vi "SwerveMain.vi"   [LabVIEW 2018]
uses:
  <vilib>/Rock Robotics/WPI/ThirdParty/Phoenix-LabVIEW/Motor Controller/Controls/CTRE_Phoenix_MotorControl_ControlMode.ctl
  <vilib>/Rock Robotics/Network Tables/NT Read Numeric Array.vi
  <vilib>/Rock Robotics/Network Tables/NT Write Numeric Array.vi
types:
  T1 = typedef "WPI_MotorControlDeviceRef.ctl" = cluster{"DeviceStatus":errorcluster, "Type":T2, "PWM":cluster{"PWM Channel":T3, "DeadBand":T4}, "CAN":cluster{"Device Number":u8, "SetOutput VI Ref":variant, "GetOutput VI Ref":variant, "Enable VI Ref":variant, "Disable VI Ref":variant, "Data":variant}, "Invert":bool, "DIO PWM":cluster{"PWM \"Enable\" Channel":T3, "DIOChannel":T5, "PWM Rate":dbl}}
  T2 = typedef "WPI_MotorControlType.ctl" = enum16{"PWM", "CAN", "DIO PWM"}
  T3 = typedef "FPGA_DIOPWMChannel.ctl" = enum8{"PWM 0", "PWM 1", "PWM 2", "PWM 3", "PWM 4", "PWM 5", "PWM 6", "PWM 7", "PWM 8", "PWM 9", "PWM MXP 0", "PWM MXP 1", "PWM MXP 2", "PWM MXP 3", "PWM MXP 4", "PWM MXP 5", "PWM MXP 6", "PWM MXP 7", "PWM MXP 8", "PWM MXP 9", "Invalid"}
  T4 = typedef "WPI_PWMDeadband.ctl" = cluster{"Name":string, "maxPositivePwm":i32, "minPositivePwm":i32, "centerPwm":i32, "maxNegativePwm":i32, "minNegativePwm":i32, "angularRange":u16}
  T5 = typedef "FPGA_DIOChannel.ctl" = enum8{"DIO 0", "DIO 1", "DIO 2", "DIO 3", "DIO 4", "DIO 5", "DIO 6", "DIO 7", "DIO 8", "DIO 9", "DIO MXP 0", "DIO MXP 1", "DIO MXP 2", "DIO MXP 3", "DIO MXP 4", "DIO MXP 5", "DIO MXP 6", "DIO MXP 7", "DIO MXP 8", "DIO MXP 9", "DIO MXP 10", "DIO MXP 11", "DIO MXP 12", "DIO MXP 13", "DIO MXP 14", "DIO MXP 15", "SPI Port CS1", "SPI Port CS2", "SPI Port CS3", "SPI Port MISO", "SPI Port MOSI", "Invalid"}
  T6 = typedef "WPI_AnalogChannelDevRef.ctl" = cluster{"DevStatus":errorcluster, "Analog Channel":T7}
  T7 = typedef "FPGA_AIChannel.ctl" = enum8{"AI 0", "AI 1", "AI 2", "AI 3", "AI MXP 0", "AI MXP 1", "AI MXP 2", "AI MXP 3", "Invalid"}
  T8 = cluster{"PhoenixMotorControlDevRef":T1, "PhoenixMotorControlDevRef":T1, "PhoenixMotorControlDevRef":T1, "PhoenixMotorControlDevRef":T1}
  T9 = typedef "CTRE_Phoenix_MotorControl_ControlMode.ctl" = u16
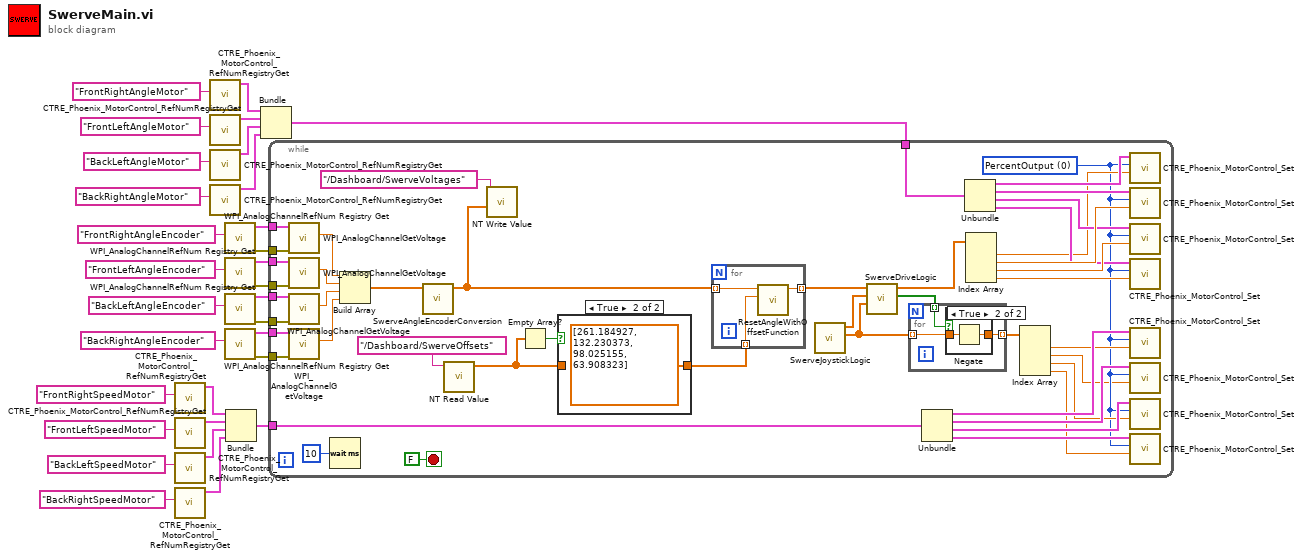
[diagram p0: block diagram]
diagram:
  n1 = call <vilib>:"CTRE_Phoenix_MotorControl_RefNumRegistryGet.vi"("refnum name"="FrontRightSpeedMotor") -> ("PhoenixMotorControlDevRef"=w8:T1)  [unwired: 9 in, 1 out]
  n2 = call <vilib>:"CTRE_Phoenix_MotorControl_RefNumRegistryGet.vi"("refnum name"="FrontLeftSpeedMotor") -> ("PhoenixMotorControlDevRef"=w16:T1)  [unwired: 9 in, 1 out]
  n3 = call <vilib>:"CTRE_Phoenix_MotorControl_RefNumRegistryGet.vi"("refnum name"="BackLeftSpeedMotor") -> ("PhoenixMotorControlDevRef"=w17:T1)  [unwired: 9 in, 1 out]
  n4 = call <vilib>:"CTRE_Phoenix_MotorControl_RefNumRegistryGet.vi"("refnum name"="BackRightSpeedMotor") -> ("PhoenixMotorControlDevRef"=w18:T1)  [unwired: 9 in, 1 out]
  n5 = call <vilib>:"CTRE_Phoenix_MotorControl_RefNumRegistryGet.vi"("refnum name"="FrontRightAngleMotor") -> ("PhoenixMotorControlDevRef"=w5:T1)  [unwired: 9 in, 1 out]
  n6 = call <vilib>:"CTRE_Phoenix_MotorControl_RefNumRegistryGet.vi"("refnum name"="FrontLeftAngleMotor") -> ("PhoenixMotorControlDevRef"=w9:T1)  [unwired: 9 in, 1 out]
  n7 = call <vilib>:"CTRE_Phoenix_MotorControl_RefNumRegistryGet.vi"("refnum name"="BackLeftAngleMotor") -> ("PhoenixMotorControlDevRef"=w10:T1)  [unwired: 9 in, 1 out]
  n8 = call <vilib>:"CTRE_Phoenix_MotorControl_RefNumRegistryGet.vi"("refnum name"="BackRightAngleMotor") -> ("PhoenixMotorControlDevRef"=w7:T1)  [unwired: 9 in, 1 out]
  n9 = call <vilib>:"WPI_AnalogChannelRefNum Registry Get.vi"("refnum name"="FrontRightAngleEncoder") -> ("error out"=w4:errorcluster, "AIDeviceRef"=w14:T6)  [unwired: 9 in]
  n10 = call <vilib>:"WPI_AnalogChannelRefNum Registry Get.vi"("refnum name"="FrontLeftAngleEncoder") -> ("error out"=w3:errorcluster, "AIDeviceRef"=w13:T6)  [unwired: 9 in]
  n11 = call <vilib>:"WPI_AnalogChannelRefNum Registry Get.vi"("refnum name"="BackLeftAngleEncoder") -> ("error out"=w2:errorcluster, "AIDeviceRef"=w12:T6)  [unwired: 9 in]
  n12 = call <vilib>:"WPI_AnalogChannelRefNum Registry Get.vi"("refnum name"="BackRightAngleEncoder") -> ("error out"=w1:errorcluster, "AIDeviceRef"=w11:T6)  [unwired: 9 in]
  n13 = Bundle("PhoenixMotorControlDevRef"=w8, "PhoenixMotorControlDevRef"=w16, "PhoenixMotorControlDevRef"=w17, "PhoenixMotorControlDevRef"=w18) -> (w15:T8)  [unwired: 1 in]
  n14 = Bundle("PhoenixMotorControlDevRef"=w5, "PhoenixMotorControlDevRef"=w9, "PhoenixMotorControlDevRef"=w10, "PhoenixMotorControlDevRef"=w7) -> (w6:T8)  [unwired: 1 in]
  n15 = while {
    tunnel: w15 -> [w56]
    tunnel: w14 -> [w43]
    tunnel: w13 -> [w38]
    tunnel: w12 -> [w35]
    tunnel: w11 -> [w41]
    tunnel: w6 -> [w55]
    tunnel: w4 -> [w44]
    tunnel: w3 -> [w37]
    tunnel: w2 -> [w34]
    tunnel: w1 -> [w40]
    stop <- FALSE stop-if-true
    w48 = T9 0 items=["PercentOutput"=0, "Position"=1, "Velocity"=2, "Current"=3, "Follower"=5, "MotionProfile"=6, "MotionMagic"=7, "MotionProfileArc"=10, "Disabled"=15] ("Control Mode")
    n16 = call <vilib>:"WPI_AnalogChannelGetVoltage.vi"("error in (no error)"=w44, "AIDeviceRef"=w43) -> ("Voltage"=w42:dbl)  [unwired: 7 in, 2 out]
    n17 = call <vilib>:"WPI_AnalogChannelGetVoltage.vi"("error in (no error)"=w37, "AIDeviceRef"=w38) -> ("Voltage"=w36:dbl)  [unwired: 7 in, 2 out]
    n18 = call <vilib>:"WPI_AnalogChannelGetVoltage.vi"("error in (no error)"=w34, "AIDeviceRef"=w35) -> ("Voltage"=w33:dbl)  [unwired: 7 in, 2 out]
    n19 = call <vilib>:"WPI_AnalogChannelGetVoltage.vi"("error in (no error)"=w40, "AIDeviceRef"=w41) -> ("Voltage"=w39:dbl)  [unwired: 7 in, 2 out]
    n20 = Wait (ms)(milliseconds to wait=u32 10) -> ()  [unwired: 1 out]
    n21 = Build Array(w42, w36, w33, w39) -> (w54:dbl[])
    n22 = call "SwerveAngleEncoderConversion.vi"("Voltages"=w54) -> ("Angles"=w53:dbl[])  [unwired: 10 in]
    n23 = call-poly <vilib>:"NT Read Value.vi"("Name"="/Dashboard/SwerveOffsets") -> ("Numeric Array"=w45:dbl[])  [unwired: 9 in, 1 out]
    n24 = call-poly <vilib>:"NT Write Value.vi"("Numeric Array"=w53, "Name"="/Dashboard/SwerveVoltages") -> ()  [unwired: 9 in, 1 out]
    n25 = Empty Array?(array=w45) -> (empty?=w47:bool)
    n26 = case shown="True" w47 {
      tunnel: [w77 dbl[] [261.184927, 132.230373, 98.025155, 63.908323]] -> w46
      tunnel: w45 -> [w77 _]
      frame False {
      }
      frame True {
      }
    }
    n27 = for {
      tunnel: w53 -> [w79] mode=indexing
      tunnel: w46 -> [w81] mode=indexing
      tunnel: [w80] -> w64 mode=indexing
      n28 = call "ResetAngleWithOffsetFunction.vi"("Offset"=w81, "AngleInput"=w79) -> ("AngleOutput"=w80:dbl)  [unwired: 9 in]
    }
    n29 = call "SwerveJoystickLogic.vi"() -> ("Speeds"=w61:dbl[], "Angles"=w63:dbl[])  [unwired: 9 in]
    n30 = call "SwerveDriveLogic.vi"("Speeds"=w61, "AngleSetpoints"=w63, "AngleEncoders"=w64) -> ("AngleMotorsReversed"=w65:bool[], "AngleMotorOutputs"=w62:dbl[])  [unwired: 7 in]
    n31 = for {
      tunnel: w61 -> [w83] mode=indexing
      tunnel: [w84] -> w70 mode=indexing
      tunnel: w65 -> [w82] mode=indexing
      n32 = case shown="True" w82 {
        tunnel: w83 -> [w85 w87]
        tunnel: [w85 w86] -> w84
        frame False {
        }
        frame True {
          n33 = Negate(x=w87) -> (-x=w86:dbl)
        }
      }
    }
    n34 = Unbundle(w56) -> ("PhoenixMotorControlDevRef"=w60:T1, "PhoenixMotorControlDevRef"=w69:T1, "PhoenixMotorControlDevRef"=w68:T1, "PhoenixMotorControlDevRef"=w67:T1)
    n35 = Unbundle(w55) -> ("PhoenixMotorControlDevRef"=w73:T1, "PhoenixMotorControlDevRef"=w72:T1, "PhoenixMotorControlDevRef"=w71:T1, "PhoenixMotorControlDevRef"=w66:T1)
    n36 = Index Array(array=w62) -> (element #1=w51:dbl, element #2=w75:dbl, element #3=w74:dbl, element #4=w52:dbl)  [unwired: 4 in]
    n37 = Index Array(array=w70) -> (element #1=w50:dbl, element #2=w31:dbl, element #3=w49:dbl, element #4=w32:dbl)  [unwired: 4 in]
    n38 = call <vilib>:"CTRE_Phoenix_MotorControl_Set.vi"("Output"=w51, "Control Mode"=w48, "PhoenixMotorControlDevRef"=w73) -> ()  [unwired: 6 in, 3 out]
    n39 = call <vilib>:"CTRE_Phoenix_MotorControl_Set.vi"("Output"=w75, "Control Mode"=w48, "PhoenixMotorControlDevRef"=w72) -> ()  [unwired: 6 in, 3 out]
    n40 = call <vilib>:"CTRE_Phoenix_MotorControl_Set.vi"("Output"=w74, "Control Mode"=w48, "PhoenixMotorControlDevRef"=w71) -> ()  [unwired: 6 in, 3 out]
    n41 = call <vilib>:"CTRE_Phoenix_MotorControl_Set.vi"("Output"=w52, "Control Mode"=w48, "PhoenixMotorControlDevRef"=w66) -> ()  [unwired: 6 in, 3 out]
    n42 = call <vilib>:"CTRE_Phoenix_MotorControl_Set.vi"("Output"=w50, "Control Mode"=w48, "PhoenixMotorControlDevRef"=w60) -> ()  [unwired: 6 in, 3 out]
    n43 = call <vilib>:"CTRE_Phoenix_MotorControl_Set.vi"("Output"=w31, "Control Mode"=w48, "PhoenixMotorControlDevRef"=w69) -> ()  [unwired: 6 in, 3 out]
    n44 = call <vilib>:"CTRE_Phoenix_MotorControl_Set.vi"("Output"=w49, "Control Mode"=w48, "PhoenixMotorControlDevRef"=w68) -> ()  [unwired: 6 in, 3 out]
    n45 = call <vilib>:"CTRE_Phoenix_MotorControl_Set.vi"("Output"=w32, "Control Mode"=w48, "PhoenixMotorControlDevRef"=w67) -> ()  [unwired: 6 in, 3 out]
  }
